vi "heartbeatRead.vi"() -> ()   [LabVIEW 2018, in "MotorControllerClass.lvclass"]
uses:
  BMS/MotorControllerClass.lvclass
  <vilib>/CANopenLib/CANOPEN.llb/CANopen Heartbeat State Read.vi
panel:
  out "MotorControllerClass out":refnum<class "MotorControllerClass.lvclass">
  in  "MotorControllerClass in":refnum<class "MotorControllerClass.lvclass">
  out "timestamp":timestamp
  out "heartbeat object out":refnum<k20>
  in  "heartbeat object in":refnum<k20>
  out "error out":errorcluster
  in  "error in (no error)":errorcluster
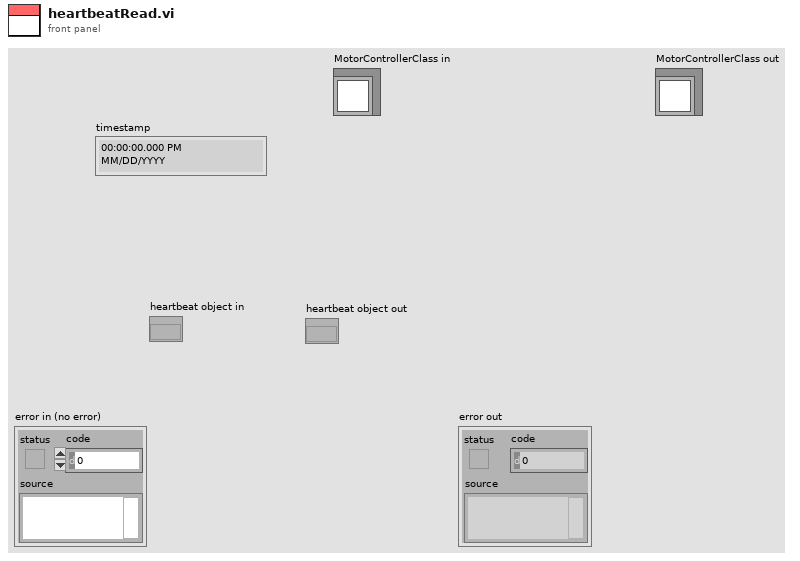
[diagram p1: front panel]
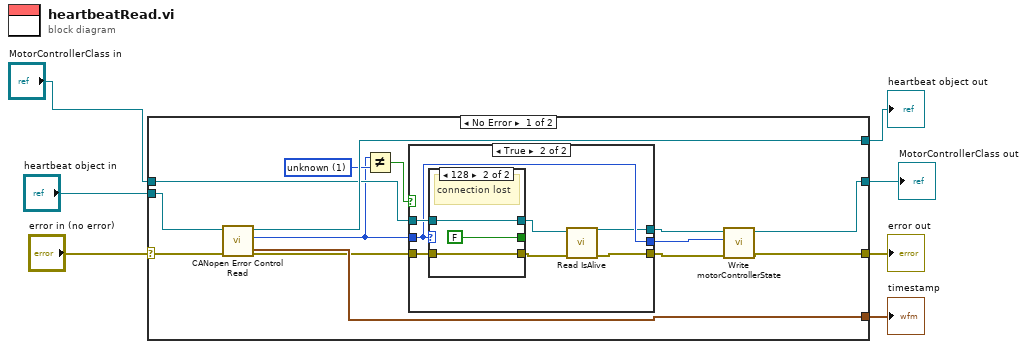
[diagram p0: block diagram]
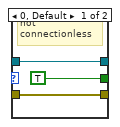
[diagram p3: hidden frame]
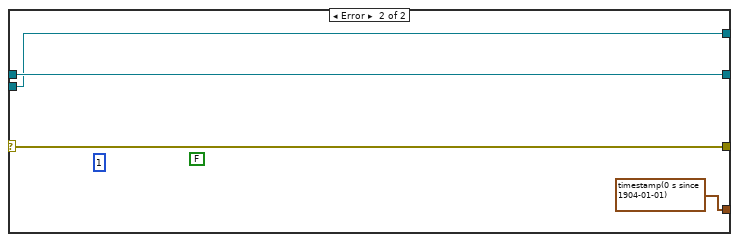
[diagram p4: hidden frame]
diagram:
  n1 = case shown="No Error" "error in (no error)" {
    selector: "error in (no error)" -> [w21 w41]
    tunnel: [w10 w41] -> w6
    tunnel: [w9 w40] -> w1
    tunnel: "MotorControllerClass in" -> [w16 w40]
    tunnel: "heartbeat object in" -> [w20 w39]
    tunnel: [w19 w39] -> w4
    tunnel: [w18 timestamp(0 s since 1904-01-01) ("timestamp")] -> w3
    frame No Error {
      w14 = u16 1 items=["unknown"=1, "bootup"=0, "stopped"=4, "operational"=5, "pre-operational"=127, "connection lost"=128] ("state")
      n2 = call-poly <vilib>:"CANopen Error Control Read.vi"("error in (no error)"=w21, "heartbeat object in"=w20) -> ("error out"=w15:errorcluster, "state"=w13:u16, "heartbeat object out"=w19:refnum<k20>, "timestamp"=w18:timestamp)  [unwired: 6 in]
      n3 = Not Equal?(x=w13, y=w14) -> (x != y?=w17:bool)
      n4 = case shown="True" w17 {
        tunnel: w16 -> [w24 w31]
        tunnel: w13 -> [w22 w29]
        tunnel: w15 -> [w23 w30]
        tunnel: [w24 w28] -> w12
        tunnel: [w23 w26] -> w11
        tunnel: [w22 w29] -> w8
        frame False {
        }
        frame True {
          n5 = case shown="128" w29 {
            tunnel: [TRUE ("isAlive") FALSE ("isAlive")] -> _
            tunnel: w31 -> [w34 w36]
            tunnel: [w34 w36] -> w25
            tunnel: w30 -> [w32 w35]
            tunnel: [w32 w35] -> w27
            frame 0, Default {
              # "not connectionless"
            }
            frame 128 {
              # "connection lost"
            }
          }
          n6 = call-dynamic "Read IsAlive.vi"("error in (no error)"=w27, "MotorControllerClass in"=w25) -> ("error out"=w26:errorcluster, "MotorControllerClass out"=w28:refnum<class "MotorControllerClass.lvclass">)  [unwired: 7 in, 1 out]
        }
      }
      n7 = call-dynamic "Write motorControllerState.vi"("error in (no error)"=w11, "motorControllerState"=w8, "MotorControllerClass in"=w12) -> ("error out"=w10:errorcluster, "MotorControllerClass out"=w9:refnum<class "MotorControllerClass.lvclass">)  [unwired: 7 in]
    }
    frame Error {
      (unwired) FALSE
      (unwired) u16 1 ("state")
    }
  }
  "error out" <- w6
  "heartbeat object out" <- w4
  "timestamp" <- w3
  "MotorControllerClass out" <- w1
